vi "Save Time to File.vi"(0 "file path (dialog if empty)":path=path "c:/data/HEWH_STATUS.csv", 5 "String":string="Startup Executed ") -> (4 "date string":string, 6 "time string":string)   [LabVIEW 2014]
uses:
  <vilib>/Utility/file.llb/Write To Spreadsheet File (string).vi
panel:
  out "date string 2":string
  out "time string 2":string
  in  "stop":bool
  in  "Reason for Startup":string="BSOD"
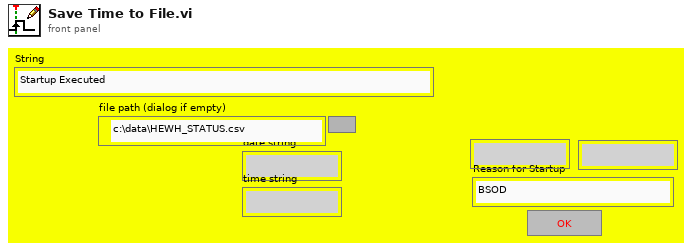
[diagram p1: front panel]
types:
  T1 = enum32{"Invalid", "Standard", "Closed", "Hidden", "Minimized", "Maximized"}
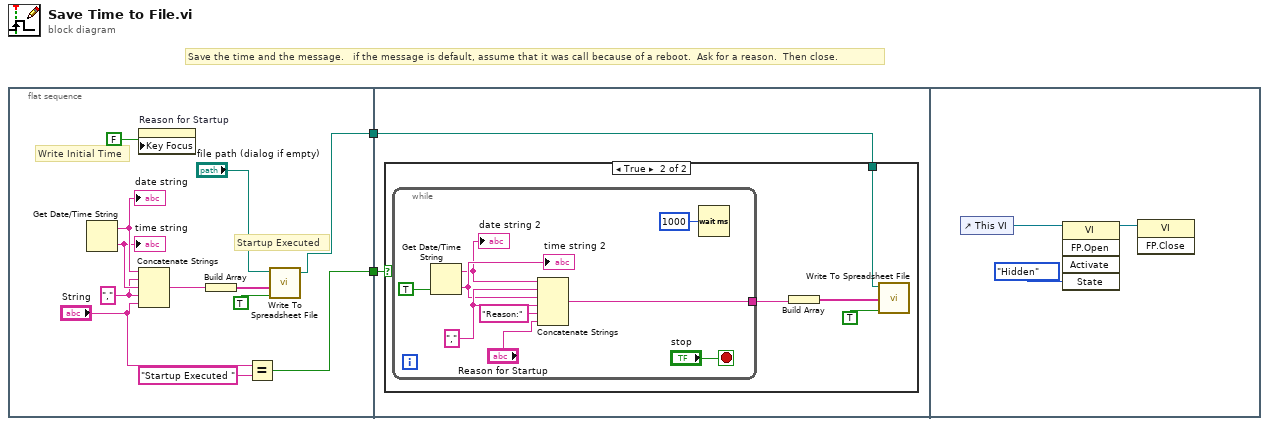
[diagram p0: block diagram]
diagram:
  # "Save the time and the message.   if the message is default, assume that it was call because of a reboot.  Ask for a reason.  Then close."
  n1 = flat-sequence {
    tunnel: [w5] -> w2
    tunnel: [w4] -> w1
    tunnel: w2 -> [w16]
    tunnel: w1 -> [w15]
    frame #0 {
      w8 = ","
      # "Startup Executed"
      # "Write Initial Time"
      n2 = Get Date/Time String() -> (date string=w14:string, time string=w13:string)  [unwired: 3 in]
      "date string" <- w14
      "time string" <- w13
      n3 = property on="Reason for Startup" class="Str"("Key Focus"=FALSE) -> ()  [unwired: 2 in, 2 out]
      n4 = Concatenate Strings(w14, w8, w13, w8, "String") -> (w12:string)
      n5 = Build Array(w12) -> (w11:string[])
      n6 = Equal?(x="String", y="Startup Executed ") -> (x = y?=w5:bool)
      n7 = call-poly <vilib>:"Write To Spreadsheet File.vi"("append to file? (new file:F)"=TRUE, "1D data"=w11, "file path (dialog if empty)"="file path (dialog if empty)") -> ("new file path (Not A Path if cancelled)"=w4:path)  [unwired: 5 in]
    }
    frame #1 {
      n8 = case shown="True" w16 {
        tunnel: w15 -> [_ w17]
        frame False {
        }
        frame True {
          n9 = while {
            tunnel: [w22] -> w19
            stop <- "stop" stop-if-true
            w27 = ","
            n10 = Get Date/Time String(want seconds? (F)=TRUE) -> (date string=w25:string, time string=w26:string)  [unwired: 2 in]
            "date string 2" <- w25
            "time string 2" <- w26
            n11 = Concatenate Strings(w25, w27, w26, w27, "Reason:" ("string"), "Reason for Startup") -> (w22:string)
            n12 = Wait (ms)(milliseconds to wait=u32 1000) -> ()  [unwired: 1 out]
          }
          n13 = Build Array(w19) -> (w18:string[])
          n14 = call-poly <vilib>:"Write To Spreadsheet File.vi"("append to file? (new file:F)"=TRUE, "1D data"=w18, "file path (dialog if empty)"=w17) -> ()  [unwired: 5 in, 1 out]
        }
      }
    }
    frame #2 {
      n15 = control-ref of="This VI"() -> (w32:refnum<vi>)
      n16 = invoke class="VI" method="FP.Open"(reference=w32, "State"=T1."Hidden") -> (reference out=w31:refnum<vi>)  [unwired: 3 in, 4 out]
      n17 = invoke class="VI" method="FP.Close"(reference=w31) -> ()  [unwired: 2 in, 3 out]
    }
  }
